vi "Configuration Keys.vi"(8 "error in":errorcluster, 11 "Chronometer in":refnum<class "Chronometer.lvclass">) -> (0 "error out":errorcluster, 2 "Required Keys":string[](array[string]), 3 "Chronometer out":refnum<class "Chronometer.lvclass">)   [LabVIEW 2023, in "Chronometer.lvlib" / "Chronometer.lvclass"]
doc: "Configuration Keys is a dynamic dispatch VI that reads a full inheritance chain's required key list.\n\nThis means each instrument must override this vi, and call the parent method . The end result is a comprehensive list of required keys that must be present in an instrument's config.ini file to correctly function."
uses:
  Chronometer.lvclass
  builds/Tools/Config.lvlibp/Config.lvclass
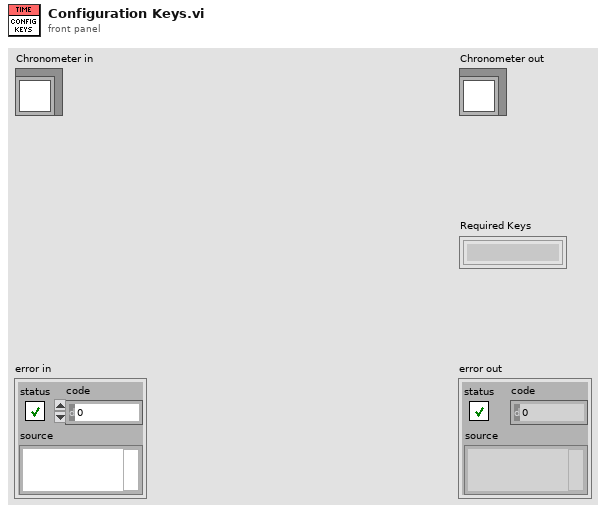
[diagram p1: front panel]
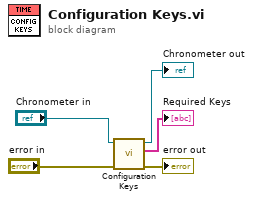
[diagram p0: block diagram]
diagram:
  n1 = call-parent "Configuration Keys.vi"("error in (no error)"="error in", "Config in"="Chronometer in") -> ("error out"=→"error out":errorcluster, "Required Keys"=→"Required Keys":string[], "Config out"=→"Chronometer out":refnum<class "Chronometer.lvclass">)  [unwired: 7 in]
